vi "Calibration key params array to key string.vi"(6 "Calibration Type":string, 7 "Pixels":cluster{"X Pixels":i32, "Y Pixels":i32}, 9 "Imaging Reso Key Parameters":T3, 10 "Imaging Galvo Key Parameters":T3, 11 "Stimulating Galvo Key Parameters":T3) -> (3 "Key String Out":string)   [LabVIEW 2012]
uses:
  Custom Controls and Typedefs/Calibration Key Param structure.ctl
  <vilib>/Utility/VariantDataType/Type.ctl
  Custom Controls and Typedefs/Galvo (Stim Path) Key Parameters.ctl
  Custom Controls and Typedefs/Galvo Key Parameters.ctl
  Custom Controls and Typedefs/Reso Key Parameters.ctl
  <vilib>/Utility/VariantDataType/VariantType.lvlib
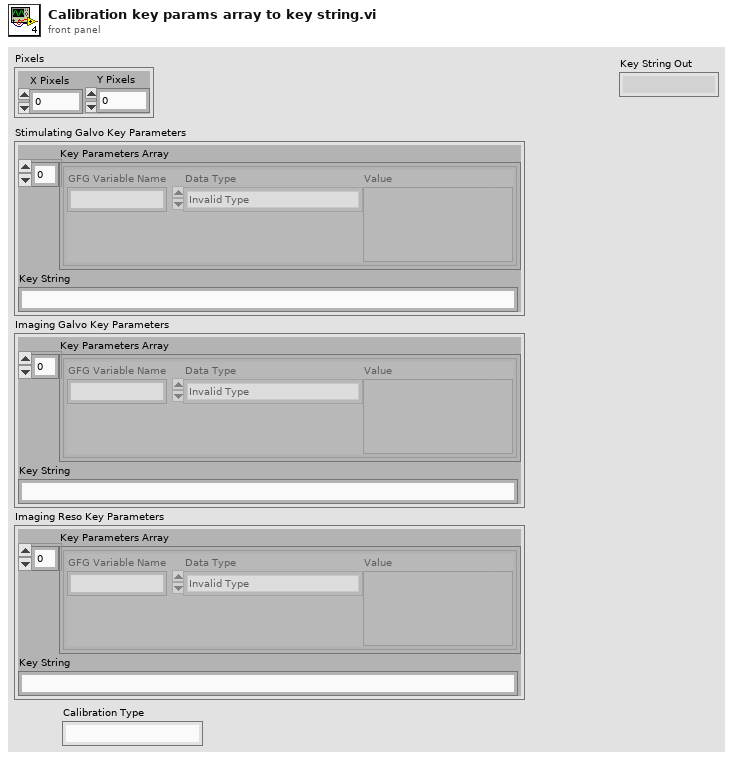
[diagram p1: front panel]
types:
  T1 = typedef "Calibration Key Param structure.ctl" = cluster{"GFG Variable Name":string, "Data Type":T2, "Value":variant}
  T2 = typedef "VariantType.lvlib/Type.ctl" = enum8{"Invalid Type", "Void", "I8", "I16", "I32", "I64", "U8", "U16", "U32", "U64", "Single Float", "Double Float", "Extended Float", "Single Complex", "Double Complex", "Extended Complex", "Enum U8", "Enum U16", "Enum U32", "Enum U64", "Single Float With Unit", "Double Float With Unit", "Extended Float With Unit", "Single Complex with Unit", "Double Complex with Unit", "Extended Complex with Unit", "Boolean", "String", "Path", "Picture", "Tag", "Array", "Cluster", "Variant", "LV Variant", "Waveform", "Timestamp", "Digital Waveform", "Digital Data", "ExpressData", "Refnum", "External Data", "VI", "Poly VI", "LabVIEW Class Instance", "Fixed Point"}
  T3 = cluster{"Key Parameters Array":T1[], "Key String":string}
  T4 = typedef "Reso Key Parameters.ctl" = T1[]
  T5 = typedef "Galvo Key Parameters.ctl" = T1[]
  T6 = typedef "Galvo (Stim Path) Key Parameters.ctl" = T1[]
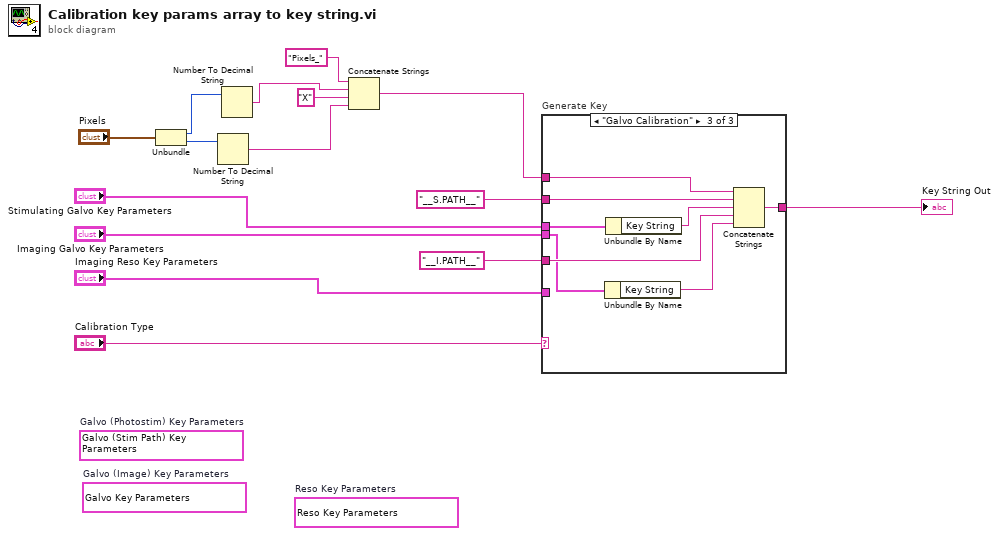
[diagram p0: block diagram]
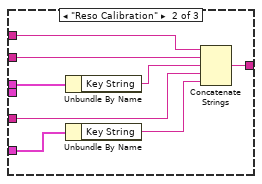
[diagram p3: hidden frame]
diagram:
  (unwired) T4 [{"GFG Variable Name"="x.voltage", "Data Type"=enum."Double Float", "Value"=variant}, {"GFG Variable Name"="y.voltage", "Data Type"=enum."Double Float", "Value"=variant}, {"GFG Variable Name"="x.correction", "Data Type"=enum."Double Float", "Value"=variant}, {"GFG Variable Name"="Start.Delay", "Data Type"=enum."Double Float", "Value"=variant}]  # Reso Key Parameters
  (unwired) T5 [{"GFG Variable Name"="x.voltage", "Data Type"=enum."Double Float", "Value"=variant}, {"GFG Variable Name"="y.voltage", "Data Type"=enum."Double Float", "Value"=variant}, {"GFG Variable Name"="x.volt.offset", "Data Type"=enum."Double Float", "Value"=variant}, {"GFG Variable Name"="y.volt.offset", "Data Type"=enum."Double Float", "Value"=variant}, {"GFG Variable Name"="Start.Delay", "Data Type"=enum."Double Float", "Value"=variant}, {"GFG Variable Name"="speed.mode", "Data Type"=enum."U16", "Value"=variant}, {"GFG Variable Name"="fill.fraction", "Data Type"=enum."Double Float", "Value"=variant}, {"GFG Variable Name"="x.bidirectional", "Data Type"=enum."Boolean", "Value"=variant}, {"GFG Variable Name"="y.bidirectional", "Data Type"=enum."Boolean", "Value"=variant}]  # Galvo (Image) Key Parameters
  (unwired) T6 [{"GFG Variable Name"="x.voltage", "Data Type"=enum."Double Float", "Value"=variant}, {"GFG Variable Name"="y.voltage", "Data Type"=enum."Double Float", "Value"=variant}, {"GFG Variable Name"="x.volt.offset", "Data Type"=enum."Double Float", "Value"=variant}, {"GFG Variable Name"="y.volt.offset", "Data Type"=enum."Double Float", "Value"=variant}]  # Galvo (Photostim) Key Parameters
  n1 = Unbundle("Pixels") -> ("X Pixels"=w14:i32, "Y Pixels"=w15:i32)
  n2 = Number To Decimal String(number=w15) -> (decimal integer string=w12:string)  [unwired: 1 in]
  n3 = Number To Decimal String(number=w14) -> (decimal integer string=w11:string)  [unwired: 1 in]
  n4 = Concatenate Strings("Pixels_" ("string"), w11, "X" ("string"), w12) -> (w3:string)
  n5 = case "Generate Key" shown="\"Galvo Calibration\"" "Calibration Type" {
    tunnel: w3 -> [_ w21 w30]
    tunnel: "Stimulating Galvo Key Parameters" -> [_ w23 w31]
    tunnel: "Imaging Galvo Key Parameters" -> [_ _ w25]
    tunnel: "Imaging Reso Key Parameters" -> [_ w22 _]
    tunnel: "__S.PATH__" ("string") -> [_ w20 w29]
    tunnel: "__I.PATH__" ("string") -> [_ w18 w27]
    tunnel: [_ w16 w24] -> w9
    frame Default {
    }
    frame "Reso Calibration" {
      n6 = Unbundle By Name(w23) -> ("Key String"=w19:string)
      n7 = Unbundle By Name(w22) -> ("Key String"=w17:string)
      n8 = Concatenate Strings(w21, w20, w19, w18, w17) -> (w16:string)
    }
    frame "Galvo Calibration" {
      n9 = Unbundle By Name(w25) -> ("Key String"=w26:string)
      n10 = Unbundle By Name(w31) -> ("Key String"=w28:string)
      n11 = Concatenate Strings(w30, w29, w28, w27, w26) -> (w24:string)
    }
  }
  "Key String Out" <- w9
